vi "Digital Read 1 Channel.vi"(8 "error in (no error)":errorcluster, 10 "Channel":i32, 11 "NI-DAQ in":refnum<class "NI-DAQ.lvclass">) -> (0 "error out":errorcluster, 2 "Value":bool=TRUE, 3 "NI-DAQ out":refnum<class "NI-DAQ.lvclass">)   [LabVIEW 2021, in "NI-DAQ.lvclass"]
uses:
  NI-DAQ.lvclass
  <vilib>/Utility/file.llb/Read Delimited Spreadsheet (string).vi
panel:
  out "index":i32
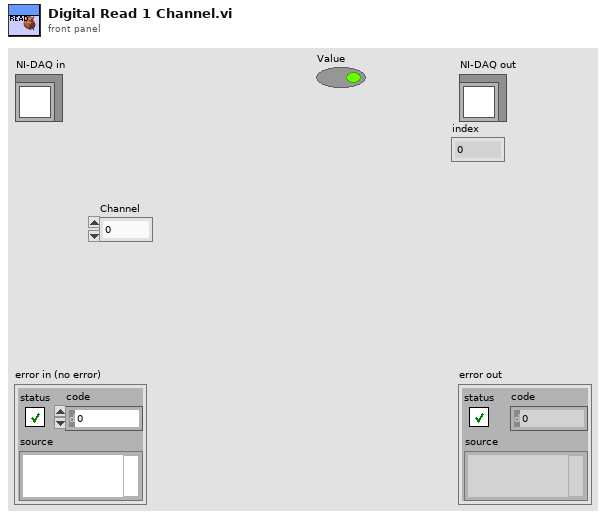
[diagram p1: front panel]
types:
  T1 = typedef "File Paths.ctl" = cluster{"Glue Pattern Folder":path, "Carrier Tray Folder":path, "Pick Up Tool Fixture Folder":path, "Components Folder":path, "Bellows Tool Offset.txt":path, "Pick Up Tool Offset.txt":path, "Dispense Tip Offset.txt":path, "Log Files":path, "Gantry Assembly Map.txt":path, "Syringe and offset map.txt":path, "Controllers Folder":path, "Local dbase config":path}
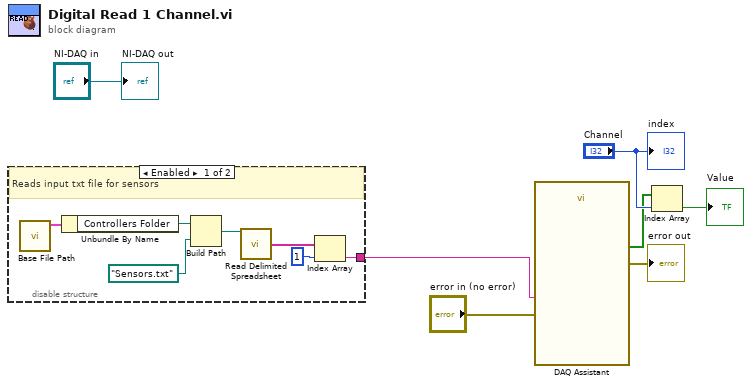
[diagram p0: block diagram]
diagram:
  n1 = disable-structure shown="Enabled" {
    disable-tunnel: [w8 _] -> w1
    frame Enabled {
      # "Reads input txt file for sensors"
      n2 = call "Base File Path.vi"() -> ("Paths Out"=w14:T1)  [unwired: 11 in]
      n3 = Unbundle By Name(w14) -> ("Controllers Folder"=w13:path)
      n4 = Build Path(base path=w13, name or relative path=path "Sensors.txt") -> (appended path=w11:path)
      n5 = call-poly <vilib>:"Read Delimited Spreadsheet.vi"("file path (dialog if empty)"=w11) -> ("first row"=w10:string[])  [unwired: 9 in, 5 out]
      n6 = Index Array(array=w10, index=1 ("dimension size")) -> (element=w8:string)
    }
    frame Disabled {
    }
  }
  n7 = call "DAQ Assistant"("error in"="error in (no error)", "device name"=w1) -> ("data"=w3:bool[], "error out"=→"error out":errorcluster)  [unwired: 15 in, 1 out]
  n8 = Index Array(array=w3, index="Channel") -> (element=→"Value":bool)
  "NI-DAQ out" <- "NI-DAQ in"
  "index" <- "Channel"
